vi "Get Probe Block.vi"() -> (2 "Probe Block":T1 {"Probe Param Array"."Sensor Block"."SensorCfgParams Array"."CalibrCoefArray" format="%#.12g"})   [LabVIEW 2015, in "Tool Cfg.lvlib"]
uses:
  Tool Cfg.lvlib
  _Probe Block Cluster--typedef.ctl
  _ProbeConfigParams Cluster--typedef.ctl
  _Sensor Block Cluster--typedef.ctl
  _SensorConfigParams Cluster--typedef.ctl
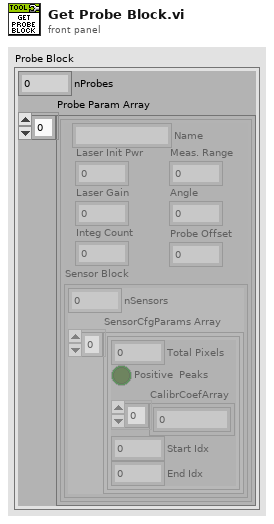
[diagram p1: front panel]
types:
  T1 = typedef "Tool Cfg.lvlib/_Probe Block Cluster--typedef.ctl" = cluster{"nProbes":u16, "Probe Param Array":T2[]}
  T2 = typedef "Tool Cfg.lvlib/_ProbeConfigParams Cluster--typedef.ctl" = cluster{"Name":string, "Laser Init Pwr":u16, "Laser Gain":u8, "Integ Count":u16, "Meas. Range":sgl, "Angle":sgl, "Probe Offset":sgl, "Sensor Block":T3}
  T3 = typedef "Tool Cfg.lvlib/_Sensor Block Cluster--typedef.ctl" = cluster{"nSensors":u16, "SensorCfgParams Array":T4[]}
  T4 = typedef "Tool Cfg.lvlib/_SensorConfigParams Cluster--typedef.ctl" = cluster{"Total Pixels":u16, "Positive  Peaks":bool, "CalibrCoefArray":dbl[], "Start Idx":u16, "End Idx":u16}
  T5 = typedef "Tool Cfg.lvlib/_Configuration Cluster_v3--typedef.ctl" = cluster{"Tool Type":u16, "Tool SN":u16, "Tool Block":T6, "Motor Block":T7, "Verification Block":T8, "Probe Block":cluster{"nProbes":u16, "Probe Param Array":T2[]}}
  T6 = typedef "Tool Cfg.lvlib/_Tool Block Cluster_v3--typedef.ctl" = cluster{"Encoder Size":u16, "Encoder Scale":u32, "Encoder Offset":i32, "MaxEncoder":i32, "MinEncoder":i32, "Start Delay":sgl, "Tool Face Ref":sgl}
  T7 = typedef "Tool Cfg.lvlib/_Motor Block Cluster_v2--typedef.ctl" = cluster{"MinMotor Speed":u16, "MaxMotor Speed":u16, "Homing Speed":u16, "Jog Speed":u16, "Inspect Speed":u16, "VBlk Speed":u16, "CleaningPos":i32, "Safe Zone":i32, "Has Motor":bool, "Use Home Index":bool}
  T8 = typedef "Tool Cfg.lvlib/_Verification Blk Cluster--typedef.ctl" = cluster{"Angle":sgl, "FlankLength1":sgl, "FlankLength2":sgl, "Location":sgl, "Serial Number":u16}
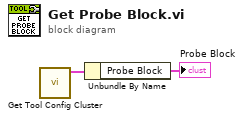
[diagram p0: block diagram]
diagram:
  n1 = call "Get Tool Config Cluster.vi"() -> ("Tool Config Cluster"=w2:T5)  [unwired: 11 in]
  n2 = Unbundle By Name(w2) -> ("Probe Block"=→"Probe Block":cluster{"nProbes":u16, "Probe Param Array":T2[]})
